vi "Read Piezo Prefocus.vi"(0 "object in":refnum<class "TBS2000Series.lvclass">, 5 "error in (no error)":errorcluster) -> (14 "object out":refnum<class "TBS2000Series.lvclass">, 15 "Frequency":dbl format="%.2p", 16 "Peak-to-Peak":dbl format="%.2p", 17 "Prefocus Channel":T1(graph), 19 "error out":errorcluster)   [LabVIEW 2023, in "TBS2000Series.lvclass"]
uses:
  TBS2000Series.lvclass
  TBS2000Series.lvclass/TBS2000Series.ctl
  <instrlib>/Tektronix TBS 2000 Series/Tektronix TBS 2000 Series.lvlib
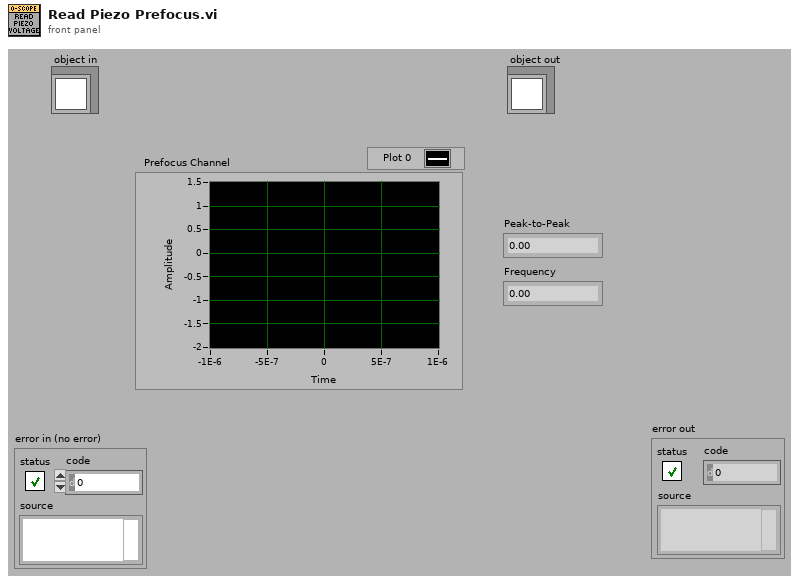
[diagram p1: front panel]
types:
  T1 = cluster{"Initial X":dbl, "X Increment":dbl, "Waveform Array":dbl[]}
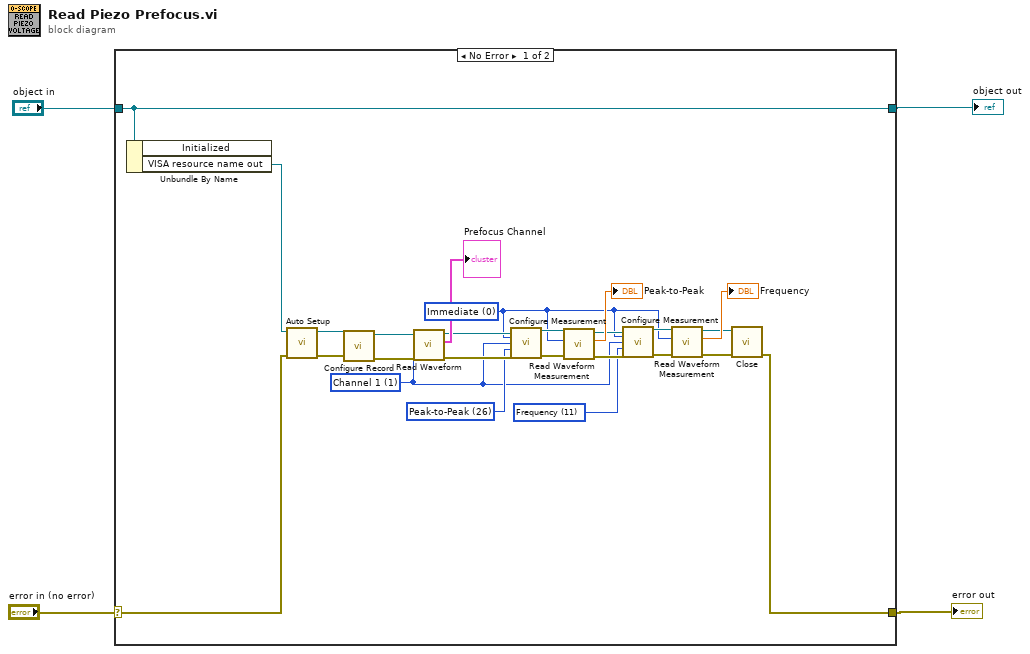
[diagram p0: block diagram]
diagram:
  n1 = case shown="No Error" "error in (no error)" {
    selector: "error in (no error)" -> [w26 w31]
    tunnel: [w5 w31] -> w1
    tunnel: [w29 w30] -> w2
    tunnel: "object in" -> [w29 w30]
    frame No Error {
      w12 = 11 items=["Amplitude", "Area", "Burst", "Cycle Area", "Cycle Mean", "Cycle RMS", "Delay RR", "Delay RF", "Delay FR", "Delay FF", "Fall Time", "Frequency", "High Reference", "Low Reference", "Max", "Mean", "Min", "- Duty Cycle", "- Edge Count", "- Overshoot", "- Pulse Count", "- Width", "+ Duty Cycle", "+ Edge Count", "Period", "Phase", "Peak-to-Peak", "+ Overshoot", "+ Pulse Count", "+ Width", "Rise", "RMS"] ("Measurement Type (30: Rise)")
      w19 = 26 items=["Amplitude", "Area", "Burst", "Cycle Area", "Cycle Mean", "Cycle RMS", "Delay RR", "Delay RF", "Delay FR", "Delay FF", "Fall Time", "Frequency", "High Reference", "Low Reference", "Max", "Mean", "Min", "- Duty Cycle", "- Edge Count", "- Overshoot", "- Pulse Count", "- Width", "+ Duty Cycle", "+ Edge Count", "Period", "Phase", "Peak-to-Peak", "+ Overshoot", "+ Pulse Count", "+ Width", "Rise", "RMS"] ("Measurement Type (30: Rise)")
      w9 = 0 items=["Immediate", "Measurement 1", "Measurement 2", "Measurement 3", "Measurement 4", "Measurement 5", "Measurement 6"] ("Measurement Slot (0: Immediate)")
      w13 = 1 items=["Math", "Channel 1", "Channel 2", "Channel 3", "Channel 4"] ("Source (1: Channel 1)")
      n2 = Unbundle By Name(w29) -> ("VISA resource name out"=w27:refnum<visa-resource-name>)  [unwired: 1 out]
      n3 = call <instrlib>:"Auto Setup.vi"("error in (no error)"=w26, "VISA resource name"=w27) -> ("error out"=w24:errorcluster, "VISA resource name out"=w25:refnum<visa-resource-name>)  [unwired: 8 in]
      n4 = call <instrlib>:"Configure Record.vi"("error in (no error)"=w24, "VISA resource name"=w25) -> ("error out"=w23:errorcluster, "VISA resource name out"=w22:refnum<visa-resource-name>)  [unwired: 8 in]
      n5 = call <instrlib>:"Read Waveform.vi"("error in (no error)"=w23, "Source (1: Channel 1)"=w13, "VISA resource name"=w22) -> ("error out"=w20:errorcluster, "Waveform Graph"=→"Prefocus Channel":T1, "VISA resource name out"=w21:refnum<visa-resource-name>)  [unwired: 6 in]
      n6 = call <instrlib>:"Configure Measurement.vi"("VISA resource name"=w21, "Measurement Slot (0: Immediate)"=w9, "Measurement Source 1 (1: Channel 1)"=w13, "Measurement Type (30: Rise)"=w19, "error in (no error)"=w20) -> ("VISA resource name out"=w18:refnum<visa-resource-name>, "error out"=w17:errorcluster)  [unwired: 9 in]
      n7 = call <instrlib>:"Read Waveform Measurement.vi"("error in (no error)"=w17, "Measurement Slot (0: Immediate)"=w9, "VISA resource name"=w18) -> ("error out"=w14:errorcluster, "Measurement"=→"Peak-to-Peak":dbl, "VISA resource name out"=w15:refnum<visa-resource-name>)  [unwired: 6 in]
      n8 = call <instrlib>:"Configure Measurement.vi"("VISA resource name"=w15, "Measurement Slot (0: Immediate)"=w9, "Measurement Source 1 (1: Channel 1)"=w13, "Measurement Type (30: Rise)"=w12, "error in (no error)"=w14) -> ("VISA resource name out"=w11:refnum<visa-resource-name>, "error out"=w10:errorcluster)  [unwired: 9 in]
      n9 = call <instrlib>:"Read Waveform Measurement.vi"("error in (no error)"=w10, "Measurement Slot (0: Immediate)"=w9, "VISA resource name"=w11) -> ("error out"=w6:errorcluster, "Measurement"=→"Frequency":dbl, "VISA resource name out"=w7:refnum<visa-resource-name>)  [unwired: 6 in]
      n10 = call <instrlib>:"Close.vi"("error in (no error)"=w6, "VISA resource name"=w7) -> ("error out"=w5:errorcluster)  [unwired: 9 in]
    }
    frame Error {
    }
  }
  "error out" <- w1
  "object out" <- w2
